vi "GUI_Create.vi"(0 "reference in":refnum<class "GUI.lvclass">, 5 "error in (no error)":errorcluster) -> (14 "reference out":refnum<class "GUI.lvclass">, 19 "error out":errorcluster)   [LabVIEW 2019]
doc: "Constructor."
uses:
  GUI.lvclass
  D:/LabASF/LabASF/src/Proccess_class/Proccess.lvclass
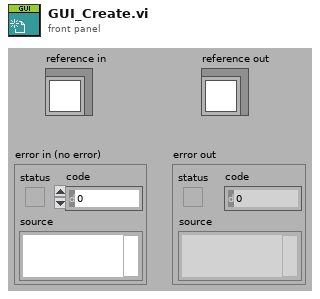
[diagram p1: front panel]
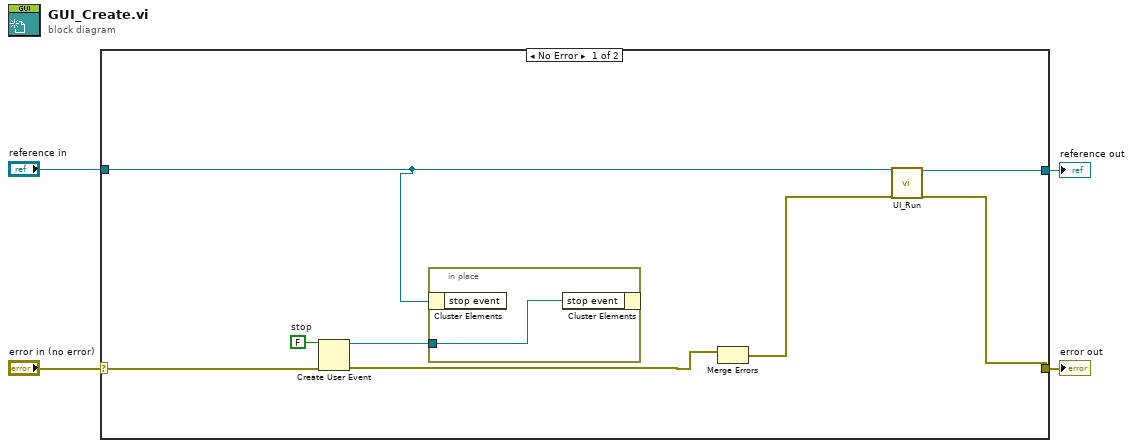
[diagram p0: block diagram]
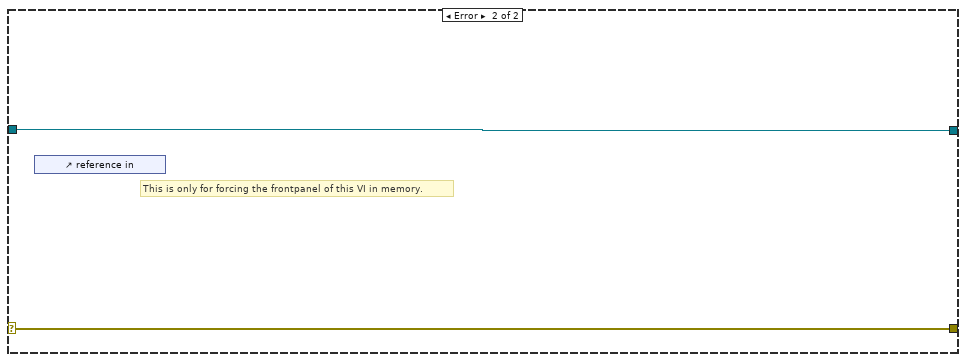
[diagram p2: hidden frame]
diagram:
  n1 = case shown="No Error" "error in (no error)" {
    selector: "error in (no error)" -> [w13 w16]
    tunnel: [w7 w16] -> w3
    tunnel: [w6 w15] -> w1
    tunnel: "reference in" -> [w5 w15]
    frame No Error {
      w9 = FALSE  # stop
      n2 = Create User Event(user event datatype=w9, error in=w13) -> (user event=w8:refnum<user-event>, error out=w12:errorcluster)
      n3 = in-place {
        in-place-border: w8 -> [w14]
        n4 = in-place-cluster #1(w5) -> ()  [unwired: 1 out]
        n5 = in-place-cluster #1("stop event"=w14) -> ()  [unwired: 1 out]
      }
      n6 = Merge Errors(w12) -> (w10:errorcluster, w11:errorcluster)
      n7 = call-dynamic "UI_Run.vi"("reference in"=w5, "error in (no error)"=w10) -> ("reference out"=w6:refnum<class "GUI.lvclass">, "error out"=w7:errorcluster)  [unwired: 16 in]
    }
    frame Error {
      # "This is only for forcing the frontpanel of this VI in memory."
      n8 = control-ref of="reference in"() -> ()  [unwired: 1 out]
    }
  }
  "error out" <- w3
  "reference out" <- w1
